vi "Launch Async.vi"   [LabVIEW 2020, in "VolatusScratch.lvlib"]
uses:
  VolatusScratch.lvlib
  TestModule/TestModule.lvclass
  C:/dev/lv20CE/relink/lv-volatus/Volatus/Module/Module.lvclass
  Volatus/Module/Module.lvclass
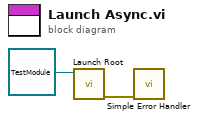
[diagram p0: block diagram]
diagram:
  n1 = call "Launch Root.vi"("Module in"=refnum<class "TestModule.lvclass"> refnum ("VolatusScratch.lvlib:TestModule.lvclass")) -> ("error out"=w1:errorcluster)  [unwired: 9 in, 1 out]
  n2 = call <vilib>:"Simple Error Handler.vi"("error in (no error)"=w1) -> ()  [unwired: 4 in, 5 out]
